vi "Find Block Statistics (SubVI).vi"(0 "Pixel Data":u8, 5 "Pixel Valid?":bool, 8 "Block Size x2":u16=8) -> (14 "Maximum":u8, 16 "Minimum":u8, 19 "Result Valid?":bool)   [LabVIEW 2014]
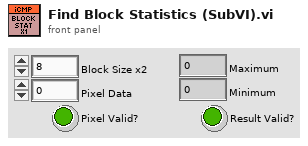
[diagram p1: front panel]
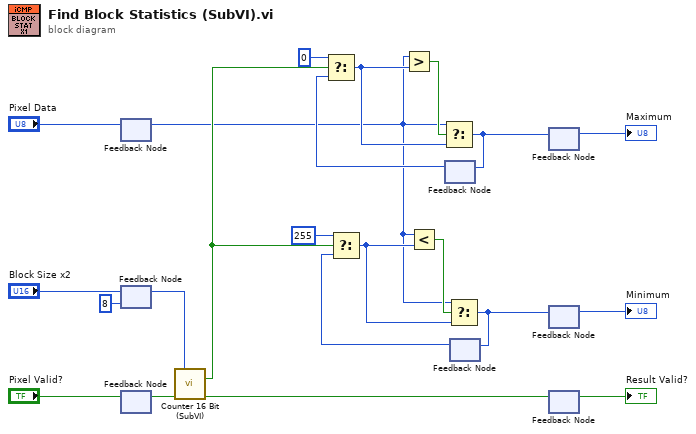
[diagram p0: block diagram]
diagram:
  n1 = feedback-in #1("Pixel Data") -> ()
  n2 = feedback #1() -> (w7:u8)  [unwired: 1 in]
  n3 = feedback-in #2("Block Size x2") -> ()
  n4 = feedback #2(u16 8 ("Block Size x2")) -> (w6:u16)
  n5 = feedback-in #3("Pixel Valid?") -> ()
  n6 = feedback #3() -> (w5:bool)  [unwired: 1 in]
  n7 = call "Counter 16 Bit (SubVI).vi"("Max. Count"=w6, "Enable"=w5) -> ("Count Begin?"=w19:bool, "Count End?"=w22:bool)  [unwired: 11 in, 1 out]
  n8 = feedback #4() -> (w14:u8)  [unwired: 1 in]
  n9 = Select(t=u8 0, s=w19, f=w14) -> (s? t:f=w9:u8)
  n10 = Greater?(x=w7, y=w9) -> (0:w12:bool)
  n11 = Select(t=w7, s=w12, f=w9) -> (s? t:f=w21:u8)
  n12 = feedback-in #4(w21) -> ()
  n13 = feedback #5() -> (w15:u8)  [unwired: 1 in]
  n14 = Select(t=u8 255, s=w19, f=w15) -> (s? t:f=w8:u8)
  n15 = Less?(x=w7, y=w8) -> (x < y?=w17:bool)
  n16 = Select(t=w7, s=w17, f=w8) -> (s? t:f=w20:u8)
  n17 = feedback-in #5(w20) -> ()
  n18 = feedback-in #6(w21) -> ()
  n19 = feedback #6() -> (→"Maximum":u8)  [unwired: 1 in]
  n20 = feedback-in #7(w20) -> ()
  n21 = feedback #7() -> (→"Minimum":u8)  [unwired: 1 in]
  n22 = feedback-in #8(w22) -> ()
  n23 = feedback #8() -> (→"Result Valid?":bool)  [unwired: 1 in]
